vi "progress_popup.vi"(7 "custom text":string, 10 "current":i32, 11 "total":i32) -> ()   [LabVIEW 2010]
panel:
  out "Slide 2":dbl(slide) caption="100 %" scale=0.0..100.0
  in  "text field":bool caption="time remaining: 0.0"
  in  "custom text":bool caption="bla"
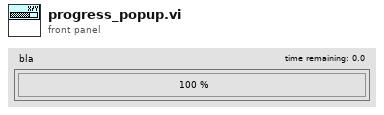
[diagram p1: front panel]
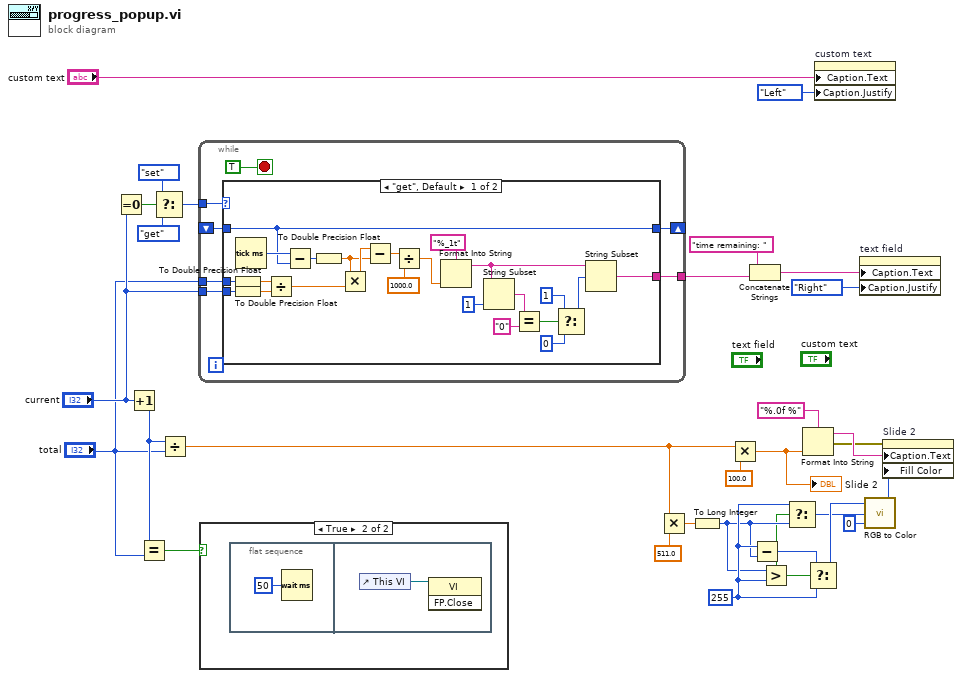
[diagram p0: block diagram]
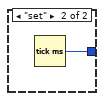
[diagram p2: hidden frame]
diagram:
  w14 = 255 ("y")
  n1 = Equal To 0?(x="current") -> (x = 0?=w25:bool)
  n2 = Increment(x="current") -> (x+1=w29:i32)
  n3 = Equal?(x=w29, y="total") -> (x = y?=w30:bool)
  n4 = Select(t=enum16{"get", "set"}."set", s=w25, f=enum16{"get", "set"}."get") -> (s? t:f=w22:enum16{"get", "set"})
  n5 = Divide(x=w29, y="total") -> (x/y=w5:dbl)
  n6 = while {
    tunnel: w22 -> [w36]
    shift-right: [w35] -> _
    shift-left: _ -> [w34]
    tunnel: "current" -> [w33]
    tunnel: "total" -> [w32]
    tunnel: [w31] -> w17
    stop <- TRUE stop-if-true
    n7 = case shown="\"get\", Default" w36 {
      tunnel: [w59 w61] -> w35
      tunnel: w34 -> [w59 _]
      tunnel: w33 -> [w58 _]
      tunnel: w32 -> [w57 _]
      tunnel: [w38 _] -> w31
      frame "get", Default {
        n8 = To Double Precision Float(number=w57) -> (double precision float=w53:dbl)
        n9 = To Double Precision Float(number=w58) -> (double precision float=w52:dbl)
        n10 = Tick Count (ms)() -> (millisecond timer value=w60:u32)
        n11 = Divide(x=w53, y=w52) -> (x/y=w56:dbl)
        n12 = Subtract(x=w60, y=w59) -> (x-y=w54:u32)
        n13 = To Double Precision Float(number=w54) -> (double precision float=w51:dbl)
        n14 = Multiply(x=w51, y=w56) -> (x*y=w55:dbl)
        n15 = Subtract(x=w55, y=w51) -> (x-y=w50:dbl)
        n16 = Divide(x=w50, y=1000.0) -> (x/y=w48:dbl)
        n17 = Format Into String(format string="%_1t", w48) -> (resulting string=w39:string)  [unwired: 2 in, 1 out]
        n18 = String Subset(string=w39, length (rest)=1 ("length (rest)")) -> (substring=w45:string)  [unwired: 1 in]
        n19 = Equal?(x=w45, y="0") -> (x = y?=w43:bool)
        n20 = Select(t=1 ("offset (0)"), s=w43, f=0) -> (s? t:f=w42:i32)
        n21 = String Subset(string=w39, offset (0)=w42) -> (substring=w38:string)  [unwired: 1 in]
      }
      frame "set" {
        n22 = Tick Count (ms)() -> (millisecond timer value=w61:u32)
      }
    }
  }
  n23 = case shown="True" w30 {
    frame False {
    }
    frame True {
      n24 = flat-sequence {
        frame #0 {
          n25 = Wait (ms)(milliseconds to wait=u32 50) -> ()  [unwired: 1 out]
        }
        frame #1 {
          n26 = control-ref of="This VI"() -> (w63:refnum<vi>)
          n27 = invoke class="VI" method="FP.Close"(reference=w63) -> ()  [unwired: 2 in, 3 out]
        }
      }
    }
  }
  n28 = Multiply(x=w5, y=511.0) -> (x*y=w12:dbl)
  n29 = To Long Integer(number=w12) -> (32bit integer=w13:i32)
  n30 = Multiply(x=w5, y=100.0) -> (x*y=w1:dbl)
  "Slide 2" <- w1
  n31 = Concatenate Strings("time remaining: " ("string"), w17) -> (w16:string)
  n32 = Subtract(x=w14, y=w13) -> (x-y=w8:i32)
  n33 = Greater?(x=w13, y=w14) -> (0:w7:bool)
  n34 = Select(t=w14, s=w7, f=w13) -> (s? t:f=w6:i32)
  n35 = Format Into String(format string="%.0f %", w1) -> (resulting string=w4:string, error out=w2:errorcluster)  [unwired: 2 in]
  n36 = Select(t=w8, s=w7, f=w14) -> (s? t:f=w10:i32)
  n37 = property on="custom text" class="Bool"("Caption.Text"="custom text", "Caption.Justify"=enum16{"Left", "Center", "Right"}."Left" ("Caption.Justification")) -> ()  [unwired: 2 in, 2 out]
  n38 = property on="text field" class="Bool"("Caption.Text"=w16, "Caption.Justify"=enum16{"Left", "Center", "Right"}."Right" ("Caption.Justification")) -> ()  [unwired: 2 in, 2 out]
  n39 = call <vilib>:"RGB to Color.vi"("B"=u8 0, "G"=w6, "R"=w10) -> ("Color"=w3:u32)
  n40 = property on="Slide 2" class="Slide (strict)"(error in=w2, "Caption.Text"=w4, "Fill Color"=w3) -> ()  [unwired: 1 in, 2 out]
